vi "MSGR Send.vi"   [LabVIEW 2018]
doc: "$Author::Richard Jennings $\n$Rev:: $\n$Date:: May, 2008 $\n\nOVERVIEW:\nReentrant VI to receive messages via a MSGR Q. If the Q does not exist this VI will create it, then wait for data.\n\nINPUTS (Controls):\n<name> - <short description of each control wired to connector pane>\n\nOUTPUTS (Indicators):\n<name> - <short description of each indicator wired to connector pane>\n\nCopyright 2008 - 2017 Jennings Embedded Servies. All rights reserved.\nAuthor makes no warranties or guarantees related to performance of the software.\nUSE AT YOUR OWN RISK\nwww.jembedded.com"
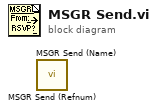
[diagram p0: block diagram]
diagram:
  n1 = call "MSGR Send (Refnum).vi"() -> ()  [unwired: 14 in, 2 out]
  n2 = call "MSGR Send (Name).vi"() -> ()  [unwired: 14 in, 2 out]
